vi "Logging.vi"(7 "Enable":bool=TRUE, 8 "error in":errorcluster, 9 "Filename":path=path "test.lvm", 10 "Array":string[](array[string]), 11 "Data":dbl[](array[numeric])) -> (0 "error out":errorcluster)   [LabVIEW 2022 SP3]
uses:
  <vilib>/express/express signal manip/GetorSetDDTAttributes/Shared VIs/TimeType.ctl
  <vilib>/express/express signal manip/GetorSetDDTAttributes/Shared VIs/TimeMode Enum to Boolean.vi
  <vilib>/express/express shared/transition.llb/Dynamic To Waveform Array.vi
  <vilib>/express/express signal manip/GetorSetDDTAttributes/Set DDT Attributes/SetT0.vi
  <vilib>/express/express signal manip/GetorSetDDTAttributes/Set DDT Attributes/sub Set StartTimeStamp.vi
  <vilib>/express/express shared/transition.llb/Waveform Array To Dynamic.vi
  <vilib>/express/express signal manip/GetorSetDDTAttributes/Set DDT Attributes/Set DDT Properties.xnode
  <vilib>/express/express signal manip/GetorSetDDTAttributes/Shared VIs/GetSetShared.lvlib
  <vilib>/express/express signal manip/GetorSetDDTAttributes/Set DDT Attributes/Set DDT Attributes.lvlib
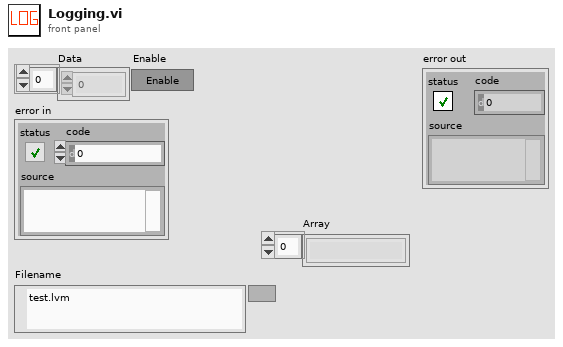
[diagram p1: front panel]
types:
  T1 = typedef "GetSetShared.lvlib/TimeType.ctl" = enum16{"Absolute", "Relative"}
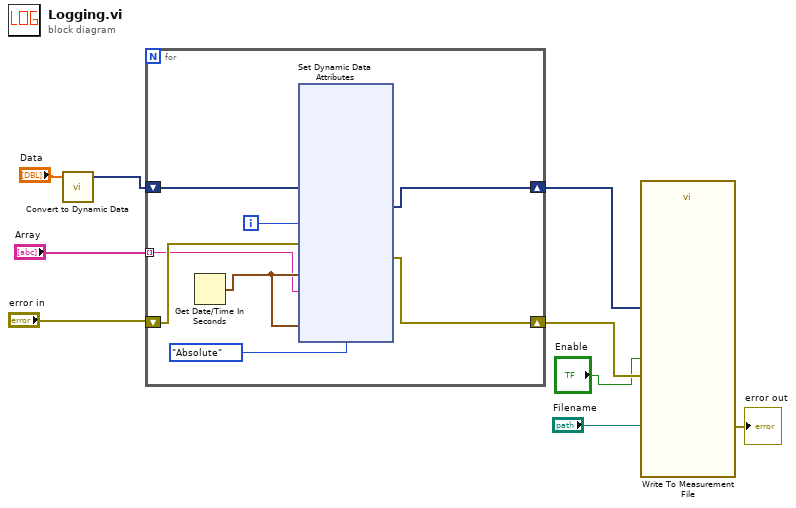
[diagram p0: block diagram]
diagram:
  n1 = call "Convert to Dynamic Data"("Array"="Data") -> ("Dynamic Data Type"=w9:dynamicdata)  [unwired: 3 in]
  n2 = for {
    shift-right: [w17] -> w5
    shift-left: w9 -> [w16]
    shift-right: [w13] -> w4
    shift-left: "error in" -> [w14]
    tunnel: "Array" -> [w10] mode=indexing
    i -> [w15]
    n3 = Get Date/Time In Seconds() -> (seconds since 1Jan1904=w12:timestamp)
    n4 = xnode "Set Dynamic Data Attributes"("Signals In"=w16, "Signal Index"=w15, "error in"=w14, "Start Timestamp"=w12, "Signal Name"=w10, "Time Mode"=TimeType."Absolute", "Timestamp"=w12) -> ("Signals Out"=w17:dynamicdata, "error out"=w13:errorcluster)
  }
  n5 = call "Write To Measurement File"("Signals"=w5, "Enable"="Enable", "error in (no error)"=w4, "Filename"="Filename") -> ("error out"=→"error out":errorcluster)  [unwired: 13 in, 2 out]
